vi "SetupTDMS.vi"(8 "error in (no error)":errorcluster, 11 "Compiled.Settings In":T1={"Name"="", "Async Init Timeout"=0, "File Data"={"Date Captured"="", "Directory"="", "Name"="", "Groups"=[], "Meta Data"=[]}, "Segment Files"=FALSE, "Segment Every"=0.0, "Trigger?"=FALSE, "Segment by"=enum."Size (MB)", "Trigger Ref"=0} {"Trigger Ref" format="%.0x"; "File Data"."Groups"."Channels"."Data Reference in" format="%.0x"}) -> (0 "error out":errorcluster, 1 "File Start Time":timestamp, 2 "tdms file out":refnum<k34>, 3 "Compiled.Settings Out":T1={"Name"="", "Async Init Timeout"=0, "File Data"={"Date Captured"="", "Directory"="", "Name"="", "Groups"=[], "Meta Data"=[]}, "Segment Files"=FALSE, "Segment Every"=0.0, "Trigger?"=FALSE, "Segment by"=enum."Size (MB)", "Trigger Ref"=0} {"Trigger Ref" format="%.0x"; "File Data"."Groups"."Channels"."Data Reference in" format="%.0x"})   [LabVIEW 2023, in "Embedded TDMS Logger Engine.lvlib"]
uses:
  Embedded TDMS Logger Engine.lvlib
  Shared/Compiled.Settings.ctl
  Shared/FileData.ctl
  Shared/GroupData.ctl
  Shared/Meta Data Item.ctl
  Shared/ChannelData.ctl
  <vilib>/NI VeriStand/Custom Device API/Data Reference.ctl
  Shared/SegmentOptions.ctl
  Shared/Embedded TDMS Logger Shared.lvlib
  <vilib>/NI VeriStand/Custom Device API/Custom Device API.lvlib
panel:
  out "path":path
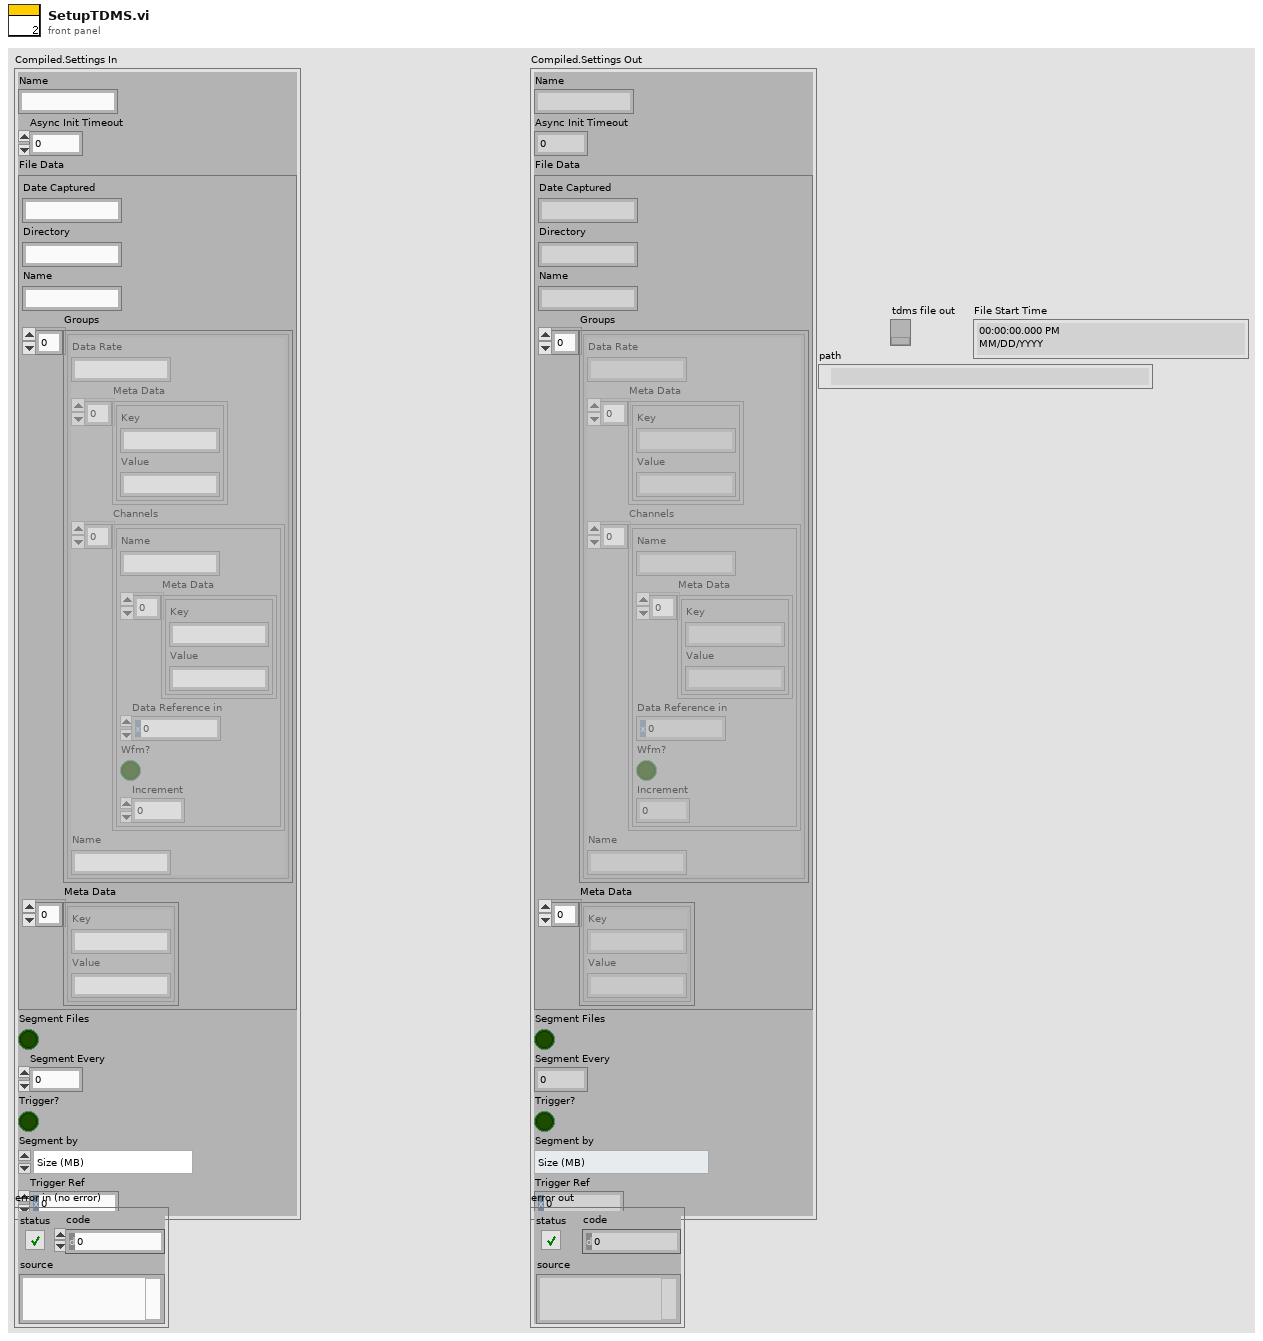
[diagram p1: front panel]
types:
  T1 = typedef "Embedded TDMS Logger Shared.lvlib/Compiled.Settings.ctl" = cluster{"Name":string, "Async Init Timeout":u16, "File Data":T2, "Segment Files":bool, "Segment Every":dbl, "Trigger?":bool, "Segment by":T7, "Trigger Ref":T6}
  T2 = typedef "Embedded TDMS Logger Shared.lvlib/FileData.ctl" = cluster{"Date Captured":string, "Directory":string, "Name":string, "Groups":T3[], "Meta Data":T4[]}
  T3 = typedef "Embedded TDMS Logger Shared.lvlib/GroupData.ctl" = cluster{"Data Rate":string, "Meta Data":T4[], "Channels":T5[], "Name":string}
  T4 = typedef "Embedded TDMS Logger Shared.lvlib/Meta Data Item.ctl" = cluster{"Key":string, "Value":string}
  T5 = typedef "Embedded TDMS Logger Shared.lvlib/ChannelData.ctl" = cluster{"Name":string, "Meta Data":T4[], "Data Reference":T6, "Wfm?":bool, "Increment":dbl}
  T6 = typedef "Custom Device API.lvlib/Data Reference.ctl" = i32
  T7 = typedef "SegmentOptions.ctl" = enum16{"Time (s)", "Size (MB)"}
  T8 = enum16{"open", "open or create", "create or replace", "create", "open (read-only)"}
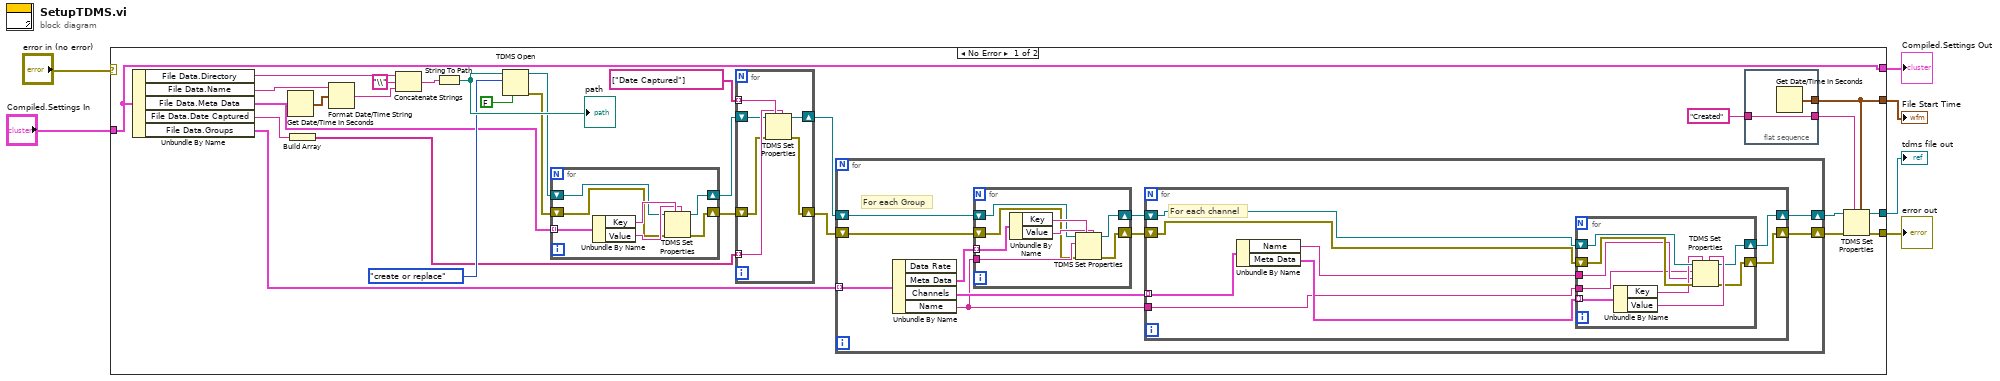
[diagram p0: block diagram]
diagram:
  n1 = case shown="No Error" "error in (no error)" {
    selector: "error in (no error)" -> [_ w85]
    tunnel: "Compiled.Settings In" -> [w13 w86]
    tunnel: [w16 w85] -> w4
    tunnel: [w15 _] -> w3
    tunnel: [w14 _] -> w2
    tunnel: [w13 w86] -> w1
    frame No Error {
      n2 = Unbundle By Name(w13) -> ("File Data.Directory"=w34:string, "File Data.Name"=w8:string, "File Data.Meta Data"=w30:T4[], "File Data.Date Captured"=w27:string, "File Data.Groups"=w7:T3[])
      n3 = Get Date/Time In Seconds() -> (seconds since 1Jan1904=w9:timestamp)
      n4 = Build Array(w27) -> (w25:string[])
      n5 = Format Date/Time String(time format string (%c)=w8, seconds (now)=w9) -> (date/time string=w10:string)  [unwired: 1 in]
      n6 = Concatenate Strings(w34, "\\" ("string"), w10) -> (w11:string)
      n7 = String To Path(string=w11) -> (path=w33:path)
      "path" <- w33
      n8 = TDMS Open(6:FALSE ("disable buffering? (T)"), 10:T8."create or replace" ("operation (0:open)"), 11:w33) -> (0:w28:errorcluster, 3:w29:refnum<k34>)  [unwired: 4 in]
      n9 = for {
        tunnel: w30 -> [w84] mode=indexing
        shift-right: [w78] -> w23
        shift-left: w28 -> [w80]
        shift-right: [w79] -> w24
        shift-left: w29 -> [w81]
        n10 = Unbundle By Name(w84) -> ("Key"=w83:string, "Value"=w82:string)
        n11 = TDMS Set Properties(5:w82, 7:w83, 8:w80, 11:w81) -> (0:w78:errorcluster, 3:w79:refnum<k34>)  [unwired: 1 in, 3 out]
      }
      n12 = for {
        tunnel: string[] ["Date Captured"] -> [w77] mode=indexing
        tunnel: w25 -> [w76] mode=indexing
        shift-right: [w72] -> w19
        shift-left: w23 -> [w74]
        shift-right: [w73] -> w20
        shift-left: w24 -> [w75]
        n13 = TDMS Set Properties(5:w76, 7:w77, 8:w74, 11:w75) -> (0:w72:errorcluster, 3:w73:refnum<k34>)  [unwired: 1 in, 3 out]
      }
      n14 = for {
        tunnel: w7 -> [w46] mode=indexing
        shift-right: [w37] -> w18
        shift-left: w20 -> [w42]
        shift-right: [w38] -> w17
        shift-left: w19 -> [w40]
        # "For each Group"
        n15 = Unbundle By Name(w46) -> ("Meta Data"=w45:T4[], "Channels"=w44:T5[], "Name"=w43:string)  [unwired: 1 out]
        n16 = for {
          tunnel: w45 -> [w71] mode=indexing
          tunnel: w43 -> [w68]
          shift-right: [w66] -> w41
          shift-left: w42 -> [w67]
          shift-right: [w64] -> w39
          shift-left: w40 -> [w65]
          n17 = Unbundle By Name(w71) -> ("Key"=w70:string, "Value"=w69:string)
          n18 = TDMS Set Properties(5:w69, 7:w70, 8:w65, 10:w68, 11:w67) -> (0:w64:errorcluster, 3:w66:refnum<k34>)  [unwired: 1 in, 2 out]
        }
        n19 = for {
          tunnel: w44 -> [w54] mode=indexing
          tunnel: w43 -> [w49]
          shift-right: [w47] -> w38
          shift-left: w39 -> [w52]
          shift-right: [w48] -> w37
          shift-left: w41 -> [w53]
          # "For each channel"
          n20 = Unbundle By Name(w54) -> ("Name"=w50:string, "Meta Data"=w51:T4[])
          n21 = for {
            shift-right: [w56] -> w48
            shift-left: w53 -> [w63]
            tunnel: w51 -> [w61] mode=indexing
            tunnel: w50 -> [w58]
            tunnel: w49 -> [w57]
            shift-right: [w55] -> w47
            shift-left: w52 -> [w62]
            n22 = Unbundle By Name(w61) -> ("Key"=w60:string, "Value"=w59:string)
            n23 = TDMS Set Properties(5:w59, 7:w60, 8:w62, 9:w58, 10:w57, 11:w63) -> (0:w55:errorcluster, 3:w56:refnum<k34>)  [unwired: 2 out]
          }
        }
      }
      n24 = flat-sequence {
        tunnel: [w36] -> w14
        tunnel: [w35] -> w22
        tunnel: "Created" ("Name") -> [w35]
        frame #0 {
          n25 = Get Date/Time In Seconds() -> (seconds since 1Jan1904=w36:timestamp)
        }
      }
      n26 = TDMS Set Properties(5:w14, 7:w22, 8:w17, 11:w18) -> (0:w16:errorcluster, 3:w15:refnum<k34>)  [unwired: 1 in, 3 out]
    }
    frame Error {
    }
  }
  "Compiled.Settings Out" <- w1
  "error out" <- w4
  "tdms file out" <- w3
  "File Start Time" <- w2
